vi "ReceiveMultipleStringsNoSemaphore.vi"(8 "error in (no error)":errorcluster, 9 "waiting time ms (-1: forever)":i32=10, 11 "queue cluster":T1) -> (0 "error out":errorcluster, 1 "new value":bool, 2 "received strings":string[](array[string]), 3 "queue cluster out":T1)   [LabVIEW 2014]
uses:
  typedefs/QueueCluster.ctl
  typedefs/clientStatus.ctl
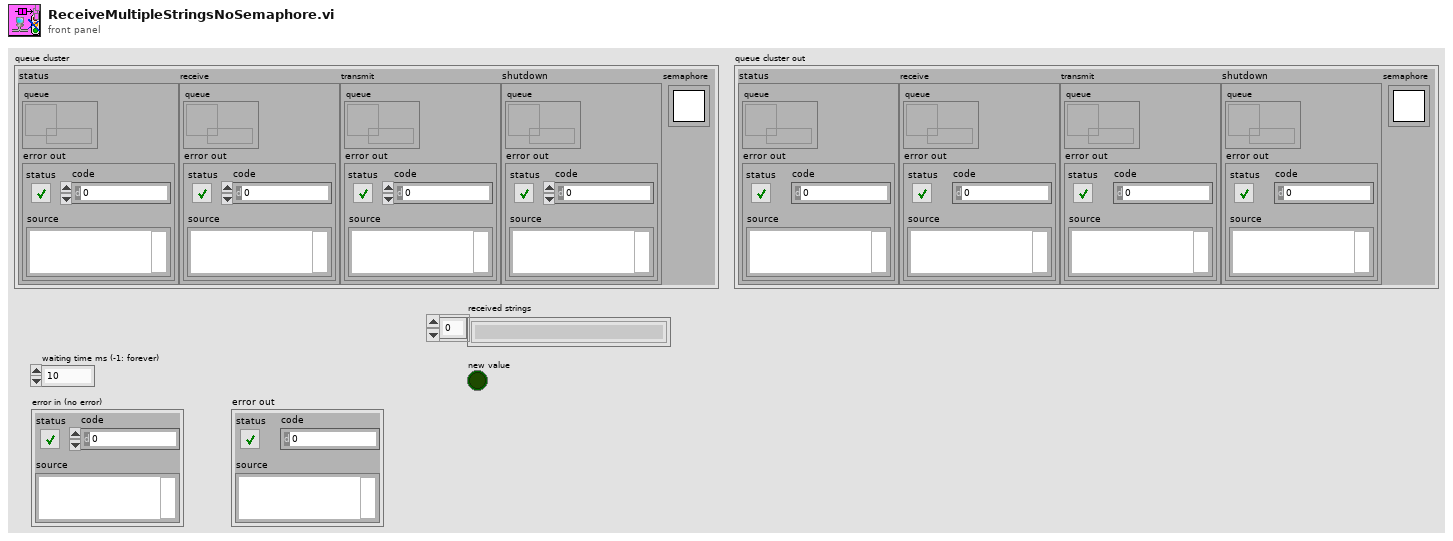
[diagram p1: front panel]
types:
  T1 = typedef "QueueCluster.ctl" = cluster{"status":cluster{"queue":refnum<queue>, "error out":errorcluster}, "receive":cluster{"queue":refnum<queue>, "error out":errorcluster}, "transmit":cluster{"queue":refnum<queue>, "error out":errorcluster}, "shutdown":cluster{"queue":refnum<queue>, "error out":errorcluster}, "semaphore":T2}
  T2 = typedef "Semaphore RefNum" = refnum<k1>
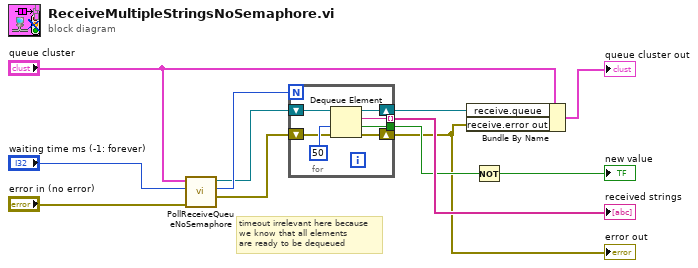
[diagram p0: block diagram]
diagram:
  # "timeout irrelevant here because\nwe know that all elements \nare ready to be dequeued"
  n1 = call "PollReceiveQueueNoSemaphore.vi"("error in (no error)"="error in (no error)", "waiting time ms (-1: forever)"="waiting time ms (-1: forever)", "queue cluster"="queue cluster") -> ("receive queue error out"=w2:errorcluster, "# elements in queue"=w4:i32, "receive queue"=w1:refnum<queue>)  [unwired: 6 in]
  n2 = for {
    N: w4 -> [_]
    tunnel: [w17] -> w8 mode=indexing
    tunnel: [w14] -> w5
    shift-right: [w19] -> w10
    shift-left: w1 -> [w18]
    shift-right: [w16] -> w3
    shift-left: w2 -> [w13]
    n3 = Dequeue Element(queue=w18, timeout in ms (-1)=50, error in (no error)=w13) -> (queue out=w19:refnum<queue>, element=w17:string, timed out?=w14:bool, error out=w16:errorcluster)
  }
  "error out" <- w3
  "received strings" <- w8
  n4 = Bundle By Name(cluster="queue cluster", "receive.queue"=w10, "receive.error out"=w3) -> (→"queue cluster out":T1)
  n5 = Not(x=w5) -> (.not. x?=→"new value":bool)
